vi "DATAreader5.vi"(6 "manual ADC rate, kHz":dbl=625.0, 7 "data info template":refnum<vi>, 10 "Cluster":cluster{"howmany":i16, "auto/man.":bool}={"howmany"=1, "auto/man."=FALSE} {"howmany" min=1 max=2}) -> (0 "error out":errorcluster, 1 "manual ADC rate?":bool, 2 "ADC type":i32, 3 "source":T1={"data path"=["D:\\LV\\testData\\11_06_14\\10_36_14ch#1", "D:\\LV\\testData\\11_06_14\\10_36_14ch#2", "D:\\LV\\testData\\11_06_14\\10_36_14ch#3", "D:\\LV\\testData\\11_06_14\\10_36_14ch#4", "D:\\LV\\testData\\11_06_14\\10_36_14ch#5", "D:\\LV\\testData\\11_06_14\\10_36_14ch#6", "D:\\LV\\testData\\11_06_14\\10_36_14ch#7", "D:\\LV\\testData\\11_06_14\\10_36_14ch#8", "D:\\LV\\testData\\11_06_14\\10_36_14ch#9", "D:\\LV\\testData\\11_06_14\\10_36_14ch#10", "D:\\LV\\testData\\11_06_14\\10_36_14ch#11", "D:\\LV\\testData\\11_06_14\\10_36_14ch#12", "D:\\LV\\testData\\11_06_14\\10_36_14ch#13", "D:\\LV\\testData\\11_06_14\\10_36_14ch#14", "D:\\LV\\testData\\11_06_14\\10_36_14ch#15", "D:\\LV\\testData\\11_06_14\\10_36_14ch#16", "D:\\LV\\testData\\11_06_14\\10_36_14ch#17", "D:\\LV\\testData\\11_06_14\\10_36_14ch#18", "D:\\LV\\testData\\11_06_14\\10_36_14ch#19", "D:\\LV\\testData\\11_06_14\\10_36_14ch#20", "D:\\LV\\testData\\11_06_14\\10_36_14ch#21", "D:\\LV\\testData\\11_06_14\\10_36_14ch#22", "D:\\LV\\testData\\11_06_14\\10_36_14ch#23", "D:\\LV\\testData\\11_06_14\\10_36_14ch#24", "D:\\LV\\testData\\11_06_14\\10_36_14ch#25", "D:\\LV\\testData\\11_06_14\\10_36_14ch#26", "D:\\LV\\testData\\11_06_14\\10_36_14ch#27", "D:\\LV\\testData\\11_06_14\\10_36_14ch#28", "D:\\LV\\testData\\11_06_14\\10_36_14ch#29", "D:\\LV\\testData\\11_06_14\\10_36_14ch#30"], "data"=[{"t0"=timestamp(0 s since 1904-01-01), "dt"=0.00015000000000000001, "Y"=array[600 elements], "attributes"=variant("source"=variant(cluster{"data path":string, "ADCintercadr_s":dbl, "data info":cluster{"probe name":string, "signal type":string, "Unit":string, "variable":string, "amplific.":dbl, "use or not *.info.txt?":i16, "U cascade, kV":string, "attenuation":dbl, "probe area, cm2":dbl, "plasma, a.m.u.":dbl}} {"data path"="D:\\LV\\testData\\11_06_14\\10_36_14ch#1", "ADCintercadr_s"=5e-06, "data info"={"probe name"="", "signal type"="", "Unit"="", "variable"="", "amplific."=0.0, "use or not *.info.txt?"=0, "U cascade, kV"="", "attenuation"=0.0, "probe area, cm2"=0.0, "plasma, a.m.u."=0.0}}))}, {"t0"=timestamp(4.999999999999959e-06 s since 1904-01-01), "dt"=0.00015000000000000001, "Y"=array[600 elements], "attributes"=variant("source"=variant(cluster{"data path":string, "ADCintercadr_s":dbl, "data info":cluster{"probe name":string, "signal type":string, "Unit":string, "variable":string, "amplific.":dbl, "use or not *.info.txt?":i16, "U cascade, kV":string, "attenuation":dbl, "probe area, cm2":dbl, "plasma, a.m.u.":dbl}} {"data path"="D:\\LV\\testData\\11_06_14\\10_36_14ch#2", "ADCintercadr_s"=5e-06, "data info"={"probe name"="", "signal type"="", "Unit"="", "variable"="", "amplific."=0.0, "use or not *.info.txt?"=0, "U cascade, kV"="", "attenuation"=0.0, "probe area, cm2"=0.0, "plasma, a.m.u."=0.0}}))}, {"t0"=timestamp(9.999999999999972e-06 s since 1904-01-01), "dt"=0.00015000000000000001, "Y"=array[600 elements], "attributes"=variant("source"=variant(cluster{"data path":string, "ADCintercadr_s":dbl, "data info":cluster{"probe name":string, "signal type":string, "Unit":string, "variable":string, "amplific.":dbl, "use or not *.info.txt?":i16, "U cascade, kV":string, "attenuation":dbl, "probe area, cm2":dbl, "plasma, a.m.u.":dbl}} {"data path"="D:\\LV\\testData\\11_06_14\\10_36_14ch#3", "ADCintercadr_s"=5e-06, "data info"={"probe name"="", "signal type"="", "Unit"="", "variable"="", "amplific."=0.0, "use or not *.info.txt?"=0, "U cascade, kV"="", "attenuation"=0.0, "probe area, cm2"=0.0, "plasma, a.m.u."=0.0}}))}, {"t0"=timestamp(1.4999999999999985e-05 s since 1904-01-01), "dt"=0.00015000000000000001, "Y"=array[600 elements], "attributes"=variant("source"=variant(cluster{"data path":string, "ADCintercadr_s":dbl, "data info":cluster{"probe name":string, "signal type":string, "Unit":string, "variable":string, "amplific.":dbl, "use or not *.info.txt?":i16, "U cascade, kV":string, "attenuation":dbl, "probe area, cm2":dbl, "plasma, a.m.u.":dbl}} {"data path"="D:\\LV\\testData\\11_06_14\\10_36_14ch#4", "ADCintercadr_s"=5e-06, "data info"={"probe name"="", "signal type"="", "Unit"="", "variable"="", "amplific."=0.0, "use or not *.info.txt?"=0, "U cascade, kV"="", "attenuation"=0.0, "probe area, cm2"=0.0, "plasma, a.m.u."=0.0}}))}, {"t0"=timestamp(1.9999999999999998e-05 s since 1904-01-01), "dt"=0.00015000000000000001, "Y"=array[600 elements], "attributes"=variant("source"=variant(cluster{"data path":string, "ADCintercadr_s":dbl, "data info":cluster{"probe name":string, "signal type":string, "Unit":string, "variable":string, "amplific.":dbl, "use or not *.info.txt?":i16, "U cascade, kV":string, "attenuation":dbl, "probe area, cm2":dbl, "plasma, a.m.u.":dbl}} {"data path"="D:\\LV\\testData\\11_06_14\\10_36_14ch#5", "ADCintercadr_s"=5e-06, "data info"={"probe name"="", "signal type"="", "Unit"="", "variable"="", "amplific."=0.0, "use or not *.info.txt?"=0, "U cascade, kV"="", "attenuation"=0.0, "probe area, cm2"=0.0, "plasma, a.m.u."=0.0}}))}, {"t0"=timestamp(2.4999999999999957e-05 s since 1904-01-01), "dt"=0.00015000000000000001, "Y"=array[600 elements], "attributes"=variant("source"=variant(cluster{"data path":string, "ADCintercadr_s":dbl, "data info":cluster{"probe name":string, "signal type":string, "Unit":string, "variable":string, "amplific.":dbl, "use or not *.info.txt?":i16, "U cascade, kV":string, "attenuation":dbl, "probe area, cm2":dbl, "plasma, a.m.u.":dbl}} {"data path"="D:\\LV\\testData\\11_06_14\\10_36_14ch#6", "ADCintercadr_s"=5e-06, "data info"={"probe name"="", "signal type"="", "Unit"="", "variable"="", "amplific."=0.0, "use or not *.info.txt?"=0, "U cascade, kV"="", "attenuation"=0.0, "probe area, cm2"=0.0, "plasma, a.m.u."=0.0}}))}, {"t0"=timestamp(2.999999999999997e-05 s since 1904-01-01), "dt"=0.00015000000000000001, "Y"=array[600 elements], "attributes"=variant("source"=variant(cluster{"data path":string, "ADCintercadr_s":dbl, "data info":cluster{"probe name":string, "signal type":string, "Unit":string, "variable":string, "amplific.":dbl, "use or not *.info.txt?":i16, "U cascade, kV":string, "attenuation":dbl, "probe area, cm2":dbl, "plasma, a.m.u.":dbl}} {"data path"="D:\\LV\\testData\\11_06_14\\10_36_14ch#7", "ADCintercadr_s"=5e-06, "data info"={"probe name"="", "signal type"="", "Unit"="", "variable"="", "amplific."=0.0, "use or not *.info.txt?"=0, "U cascade, kV"="", "attenuation"=0.0, "probe area, cm2"=0.0, "plasma, a.m.u."=0.0}}))}, {"t0"=timestamp(3.499999999999998e-05 s since 1904-01-01), "dt"=0.00015000000000000001, "Y"=array[600 elements], "attributes"=variant("source"=variant(cluster{"data path":string, "ADCintercadr_s":dbl, "data info":cluster{"probe name":string, "signal type":string, "Unit":string, "variable":string, "amplific.":dbl, "use or not *.info.txt?":i16, "U cascade, kV":string, "attenuation":dbl, "probe area, cm2":dbl, "plasma, a.m.u.":dbl}} {"data path"="D:\\LV\\testData\\11_06_14\\10_36_14ch#8", "ADCintercadr_s"=5e-06, "data info"={"probe name"="", "signal type"="", "Unit"="", "variable"="", "amplific."=0.0, "use or not *.info.txt?"=0, "U cascade, kV"="", "attenuation"=0.0, "probe area, cm2"=0.0, "plasma, a.m.u."=0.0}}))}, {"t0"=timestamp(3.9999999999999996e-05 s since 1904-01-01), "dt"=0.00015000000000000001, "Y"=array[600 elements], "attributes"=variant("source"=variant(cluster{"data path":string, "ADCintercadr_s":dbl, "data info":cluster{"probe name":string, "signal type":string, "Unit":string, "variable":string, "amplific.":dbl, "use or not *.info.txt?":i16, "U cascade, kV":string, "attenuation":dbl, "probe area, cm2":dbl, "plasma, a.m.u.":dbl}} {"data path"="D:\\LV\\testData\\11_06_14\\10_36_14ch#9", "ADCintercadr_s"=5e-06, "data info"={"probe name"="", "signal type"="", "Unit"="", "variable"="", "amplific."=0.0, "use or not *.info.txt?"=0, "U cascade, kV"="", "attenuation"=0.0, "probe area, cm2"=0.0, "plasma, a.m.u."=0.0}}))}, {"t0"=timestamp(4.4999999999999955e-05 s since 1904-01-01), "dt"=0.00015000000000000001, "Y"=array[600 elements], "attributes"=variant("source"=variant(cluster{"data path":string, "ADCintercadr_s":dbl, "data info":cluster{"probe name":string, "signal type":string, "Unit":string, "variable":string, "amplific.":dbl, "use or not *.info.txt?":i16, "U cascade, kV":string, "attenuation":dbl, "probe area, cm2":dbl, "plasma, a.m.u.":dbl}} {"data path"="D:\\LV\\testData\\11_06_14\\10_36_14ch#10", "ADCintercadr_s"=5e-06, "data info"={"probe name"="", "signal type"="", "Unit"="", "variable"="", "amplific."=0.0, "use or not *.info.txt?"=0, "U cascade, kV"="", "attenuation"=0.0, "probe area, cm2"=0.0, "plasma, a.m.u."=0.0}}))}, {"t0"=timestamp(4.999999999999997e-05 s since 1904-01-01), "dt"=0.00015000000000000001, "Y"=array[600 elements], "attributes"=variant("source"=variant(cluster{"data path":string, "ADCintercadr_s":dbl, "data info":cluster{"probe name":string, "signal type":string, "Unit":string, "variable":string, "amplific.":dbl, "use or not *.info.txt?":i16, "U cascade, kV":string, "attenuation":dbl, "probe area, cm2":dbl, "plasma, a.m.u.":dbl}} {"data path"="D:\\LV\\testData\\11_06_14\\10_36_14ch#11", "ADCintercadr_s"=5e-06, "data info"={"probe name"="", "signal type"="", "Unit"="", "variable"="", "amplific."=0.0, "use or not *.info.txt?"=0, "U cascade, kV"="", "attenuation"=0.0, "probe area, cm2"=0.0, "plasma, a.m.u."=0.0}}))}, {"t0"=timestamp(5.499999999999998e-05 s since 1904-01-01), "dt"=0.00015000000000000001, "Y"=array[600 elements], "attributes"=variant("source"=variant(cluster{"data path":string, "ADCintercadr_s":dbl, "data info":cluster{"probe name":string, "signal type":string, "Unit":string, "variable":string, "amplific.":dbl, "use or not *.info.txt?":i16, "U cascade, kV":string, "attenuation":dbl, "probe area, cm2":dbl, "plasma, a.m.u.":dbl}} {"data path"="D:\\LV\\testData\\11_06_14\\10_36_14ch#12", "ADCintercadr_s"=5e-06, "data info"={"probe name"="", "signal type"="", "Unit"="", "variable"="", "amplific."=0.0, "use or not *.info.txt?"=0, "U cascade, kV"="", "attenuation"=0.0, "probe area, cm2"=0.0, "plasma, a.m.u."=0.0}}))}, {"t0"=timestamp(5.9999999999999995e-05 s since 1904-01-01), "dt"=0.00015000000000000001, "Y"=array[600 elements], "attributes"=variant("source"=variant(cluster{"data path":string, "ADCintercadr_s":dbl, "data info":cluster{"probe name":string, "signal type":string, "Unit":string, "variable":string, "amplific.":dbl, "use or not *.info.txt?":i16, "U cascade, kV":string, "attenuation":dbl, "probe area, cm2":dbl, "plasma, a.m.u.":dbl}} {"data path"="D:\\LV\\testData\\11_06_14\\10_36_14ch#13", "ADCintercadr_s"=5e-06, "data info"={"probe name"="", "signal type"="", "Unit"="", "variable"="", "amplific."=0.0, "use or not *.info.txt?"=0, "U cascade, kV"="", "attenuation"=0.0, "probe area, cm2"=0.0, "plasma, a.m.u."=0.0}}))}, {"t0"=timestamp(6.500000000000001e-05 s since 1904-01-01), "dt"=0.00015000000000000001, "Y"=array[600 elements], "attributes"=variant("source"=variant(cluster{"data path":string, "ADCintercadr_s":dbl, "data info":cluster{"probe name":string, "signal type":string, "Unit":string, "variable":string, "amplific.":dbl, "use or not *.info.txt?":i16, "U cascade, kV":string, "attenuation":dbl, "probe area, cm2":dbl, "plasma, a.m.u.":dbl}} {"data path"="D:\\LV\\testData\\11_06_14\\10_36_14ch#14", "ADCintercadr_s"=5e-06, "data info"={"probe name"="", "signal type"="", "Unit"="", "variable"="", "amplific."=0.0, "use or not *.info.txt?"=0, "U cascade, kV"="", "attenuation"=0.0, "probe area, cm2"=0.0, "plasma, a.m.u."=0.0}}))}, {"t0"=timestamp(6.999999999999997e-05 s since 1904-01-01), "dt"=0.00015000000000000001, "Y"=array[600 elements], "attributes"=variant("source"=variant(cluster{"data path":string, "ADCintercadr_s":dbl, "data info":cluster{"probe name":string, "signal type":string, "Unit":string, "variable":string, "amplific.":dbl, "use or not *.info.txt?":i16, "U cascade, kV":string, "attenuation":dbl, "probe area, cm2":dbl, "plasma, a.m.u.":dbl}} {"data path"="D:\\LV\\testData\\11_06_14\\10_36_14ch#15", "ADCintercadr_s"=5e-06, "data info"={"probe name"="", "signal type"="", "Unit"="", "variable"="", "amplific."=0.0, "use or not *.info.txt?"=0, "U cascade, kV"="", "attenuation"=0.0, "probe area, cm2"=0.0, "plasma, a.m.u."=0.0}}))}, {"t0"=timestamp(7.499999999999998e-05 s since 1904-01-01), "dt"=0.00015000000000000001, "Y"=array[600 elements], "attributes"=variant("source"=variant(cluster{"data path":string, "ADCintercadr_s":dbl, "data info":cluster{"probe name":string, "signal type":string, "Unit":string, "variable":string, "amplific.":dbl, "use or not *.info.txt?":i16, "U cascade, kV":string, "attenuation":dbl, "probe area, cm2":dbl, "plasma, a.m.u.":dbl}} {"data path"="D:\\LV\\testData\\11_06_14\\10_36_14ch#16", "ADCintercadr_s"=5e-06, "data info"={"probe name"="", "signal type"="", "Unit"="", "variable"="", "amplific."=0.0, "use or not *.info.txt?"=0, "U cascade, kV"="", "attenuation"=0.0, "probe area, cm2"=0.0, "plasma, a.m.u."=0.0}}))}, {"t0"=timestamp(7.999999999999999e-05 s since 1904-01-01), "dt"=0.00015000000000000001, "Y"=array[600 elements], "attributes"=variant("source"=variant(cluster{"data path":string, "ADCintercadr_s":dbl, "data info":cluster{"probe name":string, "signal type":string, "Unit":string, "variable":string, "amplific.":dbl, "use or not *.info.txt?":i16, "U cascade, kV":string, "attenuation":dbl, "probe area, cm2":dbl, "plasma, a.m.u.":dbl}} {"data path"="D:\\LV\\testData\\11_06_14\\10_36_14ch#17", "ADCintercadr_s"=5e-06, "data info"={"probe name"="", "signal type"="", "Unit"="", "variable"="", "amplific."=0.0, "use or not *.info.txt?"=0, "U cascade, kV"="", "attenuation"=0.0, "probe area, cm2"=0.0, "plasma, a.m.u."=0.0}}))}, {"t0"=timestamp(8.5e-05 s since 1904-01-01), "dt"=0.00015000000000000001, "Y"=array[600 elements], "attributes"=variant("source"=variant(cluster{"data path":string, "ADCintercadr_s":dbl, "data info":cluster{"probe name":string, "signal type":string, "Unit":string, "variable":string, "amplific.":dbl, "use or not *.info.txt?":i16, "U cascade, kV":string, "attenuation":dbl, "probe area, cm2":dbl, "plasma, a.m.u.":dbl}} {"data path"="D:\\LV\\testData\\11_06_14\\10_36_14ch#18", "ADCintercadr_s"=5e-06, "data info"={"probe name"="", "signal type"="", "Unit"="", "variable"="", "amplific."=0.0, "use or not *.info.txt?"=0, "U cascade, kV"="", "attenuation"=0.0, "probe area, cm2"=0.0, "plasma, a.m.u."=0.0}}))}, {"t0"=timestamp(8.999999999999997e-05 s since 1904-01-01), "dt"=0.00015000000000000001, "Y"=array[600 elements], "attributes"=variant("source"=variant(cluster{"data path":string, "ADCintercadr_s":dbl, "data info":cluster{"probe name":string, "signal type":string, "Unit":string, "variable":string, "amplific.":dbl, "use or not *.info.txt?":i16, "U cascade, kV":string, "attenuation":dbl, "probe area, cm2":dbl, "plasma, a.m.u.":dbl}} {"data path"="D:\\LV\\testData\\11_06_14\\10_36_14ch#19", "ADCintercadr_s"=5e-06, "data info"={"probe name"="", "signal type"="", "Unit"="", "variable"="", "amplific."=0.0, "use or not *.info.txt?"=0, "U cascade, kV"="", "attenuation"=0.0, "probe area, cm2"=0.0, "plasma, a.m.u."=0.0}}))}, {"t0"=timestamp(9.499999999999998e-05 s since 1904-01-01), "dt"=0.00015000000000000001, "Y"=array[600 elements], "attributes"=variant("source"=variant(cluster{"data path":string, "ADCintercadr_s":dbl, "data info":cluster{"probe name":string, "signal type":string, "Unit":string, "variable":string, "amplific.":dbl, "use or not *.info.txt?":i16, "U cascade, kV":string, "attenuation":dbl, "probe area, cm2":dbl, "plasma, a.m.u.":dbl}} {"data path"="D:\\LV\\testData\\11_06_14\\10_36_14ch#20", "ADCintercadr_s"=5e-06, "data info"={"probe name"="", "signal type"="", "Unit"="", "variable"="", "amplific."=0.0, "use or not *.info.txt?"=0, "U cascade, kV"="", "attenuation"=0.0, "probe area, cm2"=0.0, "plasma, a.m.u."=0.0}}))}, {"t0"=timestamp(9.999999999999999e-05 s since 1904-01-01), "dt"=0.00015000000000000001, "Y"=array[600 elements], "attributes"=variant("source"=variant(cluster{"data path":string, "ADCintercadr_s":dbl, "data info":cluster{"probe name":string, "signal type":string, "Unit":string, "variable":string, "amplific.":dbl, "use or not *.info.txt?":i16, "U cascade, kV":string, "attenuation":dbl, "probe area, cm2":dbl, "plasma, a.m.u.":dbl}} {"data path"="D:\\LV\\testData\\11_06_14\\10_36_14ch#21", "ADCintercadr_s"=5e-06, "data info"={"probe name"="", "signal type"="", "Unit"="", "variable"="", "amplific."=0.0, "use or not *.info.txt?"=0, "U cascade, kV"="", "attenuation"=0.0, "probe area, cm2"=0.0, "plasma, a.m.u."=0.0}}))}, {"t0"=timestamp(0.000105 s since 1904-01-01), "dt"=0.00015000000000000001, "Y"=array[600 elements], "attributes"=variant("source"=variant(cluster{"data path":string, "ADCintercadr_s":dbl, "data info":cluster{"probe name":string, "signal type":string, "Unit":string, "variable":string, "amplific.":dbl, "use or not *.info.txt?":i16, "U cascade, kV":string, "attenuation":dbl, "probe area, cm2":dbl, "plasma, a.m.u.":dbl}} {"data path"="D:\\LV\\testData\\11_06_14\\10_36_14ch#22", "ADCintercadr_s"=5e-06, "data info"={"probe name"="", "signal type"="", "Unit"="", "variable"="", "amplific."=0.0, "use or not *.info.txt?"=0, "U cascade, kV"="", "attenuation"=0.0, "probe area, cm2"=0.0, "plasma, a.m.u."=0.0}}))}, {"t0"=timestamp(0.00010999999999999996 s since 1904-01-01), "dt"=0.00015000000000000001, "Y"=array[600 elements], "attributes"=variant("source"=variant(cluster{"data path":string, "ADCintercadr_s":dbl, "data info":cluster{"probe name":string, "signal type":string, "Unit":string, "variable":string, "amplific.":dbl, "use or not *.info.txt?":i16, "U cascade, kV":string, "attenuation":dbl, "probe area, cm2":dbl, "plasma, a.m.u.":dbl}} {"data path"="D:\\LV\\testData\\11_06_14\\10_36_14ch#23", "ADCintercadr_s"=5e-06, "data info"={"probe name"="", "signal type"="", "Unit"="", "variable"="", "amplific."=0.0, "use or not *.info.txt?"=0, "U cascade, kV"="", "attenuation"=0.0, "probe area, cm2"=0.0, "plasma, a.m.u."=0.0}}))}, {"t0"=timestamp(0.00011499999999999998 s since 1904-01-01), "dt"=0.00015000000000000001, "Y"=array[600 elements], "attributes"=variant("source"=variant(cluster{"data path":string, "ADCintercadr_s":dbl, "data info":cluster{"probe name":string, "signal type":string, "Unit":string, "variable":string, "amplific.":dbl, "use or not *.info.txt?":i16, "U cascade, kV":string, "attenuation":dbl, "probe area, cm2":dbl, "plasma, a.m.u.":dbl}} {"data path"="D:\\LV\\testData\\11_06_14\\10_36_14ch#24", "ADCintercadr_s"=5e-06, "data info"={"probe name"="", "signal type"="", "Unit"="", "variable"="", "amplific."=0.0, "use or not *.info.txt?"=0, "U cascade, kV"="", "attenuation"=0.0, "probe area, cm2"=0.0, "plasma, a.m.u."=0.0}}))}, {"t0"=timestamp(0.00011999999999999999 s since 1904-01-01), "dt"=0.00015000000000000001, "Y"=array[600 elements], "attributes"=variant("source"=variant(cluster{"data path":string, "ADCintercadr_s":dbl, "data info":cluster{"probe name":string, "signal type":string, "Unit":string, "variable":string, "amplific.":dbl, "use or not *.info.txt?":i16, "U cascade, kV":string, "attenuation":dbl, "probe area, cm2":dbl, "plasma, a.m.u.":dbl}} {"data path"="D:\\LV\\testData\\11_06_14\\10_36_14ch#25", "ADCintercadr_s"=5e-06, "data info"={"probe name"="", "signal type"="", "Unit"="", "variable"="", "amplific."=0.0, "use or not *.info.txt?"=0, "U cascade, kV"="", "attenuation"=0.0, "probe area, cm2"=0.0, "plasma, a.m.u."=0.0}}))}, {"t0"=timestamp(0.000125 s since 1904-01-01), "dt"=0.00015000000000000001, "Y"=array[600 elements], "attributes"=variant("source"=variant(cluster{"data path":string, "ADCintercadr_s":dbl, "data info":cluster{"probe name":string, "signal type":string, "Unit":string, "variable":string, "amplific.":dbl, "use or not *.info.txt?":i16, "U cascade, kV":string, "attenuation":dbl, "probe area, cm2":dbl, "plasma, a.m.u.":dbl}} {"data path"="D:\\LV\\testData\\11_06_14\\10_36_14ch#26", "ADCintercadr_s"=5e-06, "data info"={"probe name"="", "signal type"="", "Unit"="", "variable"="", "amplific."=0.0, "use or not *.info.txt?"=0, "U cascade, kV"="", "attenuation"=0.0, "probe area, cm2"=0.0, "plasma, a.m.u."=0.0}}))}, {"t0"=timestamp(0.00013000000000000002 s since 1904-01-01), "dt"=0.00015000000000000001, "Y"=array[600 elements], "attributes"=variant("source"=variant(cluster{"data path":string, "ADCintercadr_s":dbl, "data info":cluster{"probe name":string, "signal type":string, "Unit":string, "variable":string, "amplific.":dbl, "use or not *.info.txt?":i16, "U cascade, kV":string, "attenuation":dbl, "probe area, cm2":dbl, "plasma, a.m.u.":dbl}} {"data path"="D:\\LV\\testData\\11_06_14\\10_36_14ch#27", "ADCintercadr_s"=5e-06, "data info"={"probe name"="", "signal type"="", "Unit"="", "variable"="", "amplific."=0.0, "use or not *.info.txt?"=0, "U cascade, kV"="", "attenuation"=0.0, "probe area, cm2"=0.0, "plasma, a.m.u."=0.0}}))}, {"t0"=timestamp(0.00013499999999999997 s since 1904-01-01), "dt"=0.00015000000000000001, "Y"=array[600 elements], "attributes"=variant("source"=variant(cluster{"data path":string, "ADCintercadr_s":dbl, "data info":cluster{"probe name":string, "signal type":string, "Unit":string, "variable":string, "amplific.":dbl, "use or not *.info.txt?":i16, "U cascade, kV":string, "attenuation":dbl, "probe area, cm2":dbl, "plasma, a.m.u.":dbl}} {"data path"="D:\\LV\\testData\\11_06_14\\10_36_14ch#28", "ADCintercadr_s"=5e-06, "data info"={"probe name"="", "signal type"="", "Unit"="", "variable"="", "amplific."=0.0, "use or not *.info.txt?"=0, "U cascade, kV"="", "attenuation"=0.0, "probe area, cm2"=0.0, "plasma, a.m.u."=0.0}}))}, {"t0"=timestamp(0.00014 s since 1904-01-01), "dt"=0.00015000000000000001, "Y"=array[600 elements], "attributes"=variant("source"=variant(cluster{"data path":string, "ADCintercadr_s":dbl, "data info":cluster{"probe name":string, "signal type":string, "Unit":string, "variable":string, "amplific.":dbl, "use or not *.info.txt?":i16, "U cascade, kV":string, "attenuation":dbl, "probe area, cm2":dbl, "plasma, a.m.u.":dbl}} {"data path"="D:\\LV\\testData\\11_06_14\\10_36_14ch#29", "ADCintercadr_s"=5e-06, "data info"={"probe name"="", "signal type"="", "Unit"="", "variable"="", "amplific."=0.0, "use or not *.info.txt?"=0, "U cascade, kV"="", "attenuation"=0.0, "probe area, cm2"=0.0, "plasma, a.m.u."=0.0}}))}, {"t0"=timestamp(0.000145 s since 1904-01-01), "dt"=0.00015000000000000001, "Y"=array[600 elements], "attributes"=variant("source"=variant(cluster{"data path":string, "ADCintercadr_s":dbl, "data info":cluster{"probe name":string, "signal type":string, "Unit":string, "variable":string, "amplific.":dbl, "use or not *.info.txt?":i16, "U cascade, kV":string, "attenuation":dbl, "probe area, cm2":dbl, "plasma, a.m.u.":dbl}} {"data path"="D:\\LV\\testData\\11_06_14\\10_36_14ch#30", "ADCintercadr_s"=5e-06, "data info"={"probe name"="", "signal type"="", "Unit"="", "variable"="", "amplific."=0.0, "use or not *.info.txt?"=0, "U cascade, kV"="", "attenuation"=0.0, "probe area, cm2"=0.0, "plasma, a.m.u."=0.0}}))}]}, 4 "chan.in.files":i16[](array[numeric]), 11 "ADC gain applied from *.par":bool)   [LabVIEW 2014]
uses:
  <vilib>/Waveform/WDTOps.llb/WDT Number of Waveform Samples DBL.vi
panel:
  out "txt data rate":dbl[](array[numeric])
  out "allpathes":path[](array[path])
  out "Array":string[](array[string])
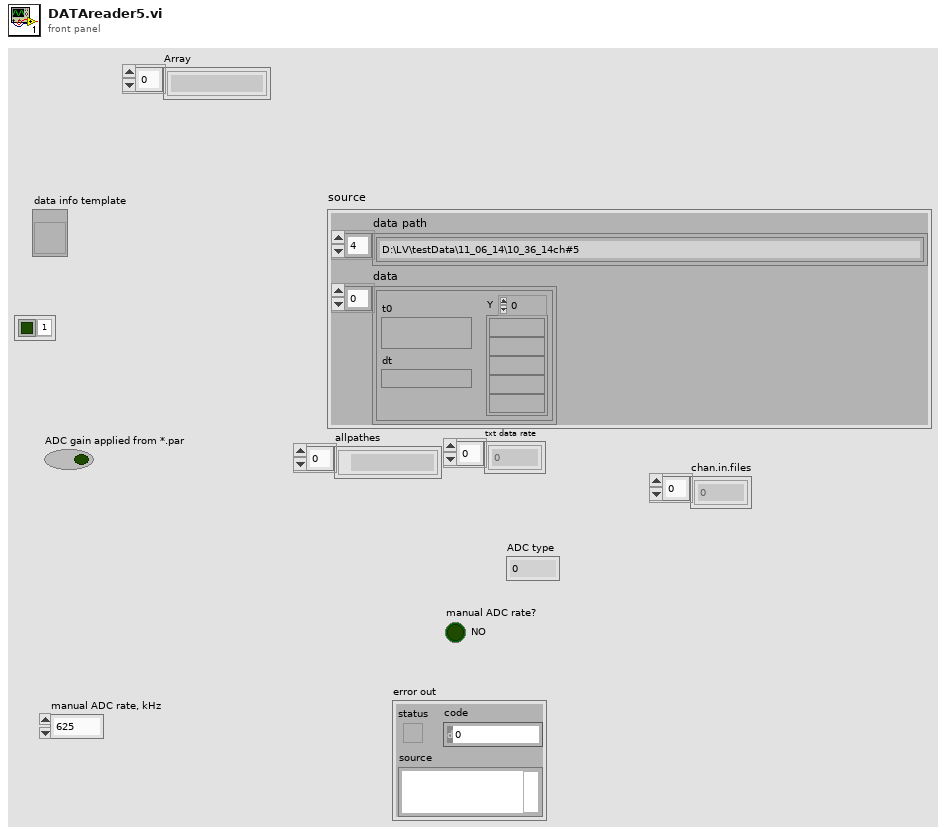
[diagram p1: front panel]
types:
  T1 = cluster{"data path":string[], "data":waveform(dbl)[]}
  T2 = enum16{"open", "replace", "create", "open or create", "replace or create", "replace or create with confirmation"}
  T3 = enum16{"deny read/write", "deny write-only", "deny none"}
  T4 = enum16{"big-endian, network order", "native, host order", "little-endian"}
  T5 = cluster{" CodeString":string, "DeviceName":string, "TimeString":string, "ChannelsMax":i16, "RealChannelsQuantity":i16, "RealKadrsQuantity":i64, "RealSamplesQuantity":i64, "TotalTime (sec) - long double in new *.par !!":string, "AdcRate (kHz)":dbl, "InterkadrDelay (ms)":dbl, "ChannelRate (kHz)":dbl, "ActiveAdcChannelArray":u32[], "AdcChannelArray":u8[], "AdcGainArray":u8[], "IsSignalArray":u8[], "DataFormat":i32, "RealKadrs64":i64, "AdcScale":dbl[], "AdcOffset":dbl[], "channel_name":string[], "LastModified":string}
  T6 = cluster{"data path":string, "ADCintercadr_s":dbl, "data info":cluster{"use or not *.info.txt?":i16, "probe name":string, "signal type":string, "Unit":string, "variable":string, "attenuation factor":dbl, "amplification factor":dbl, "extracoef#1":dbl, "extracoef#2":dbl, "U cascade, kV":string, "probe area, cm2":dbl, "plasma, a.m.u.":dbl}, "channel_name":string, "channels_in_file":i32, "LastModified":string}
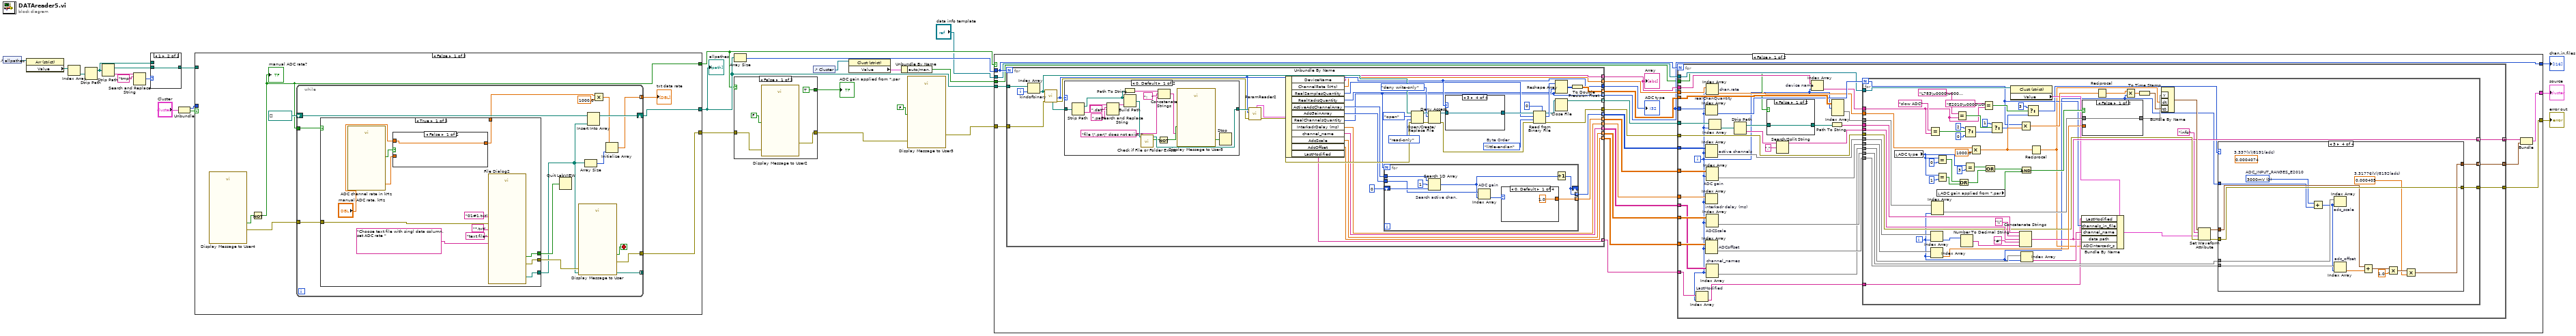
[diagram p0: block diagram]
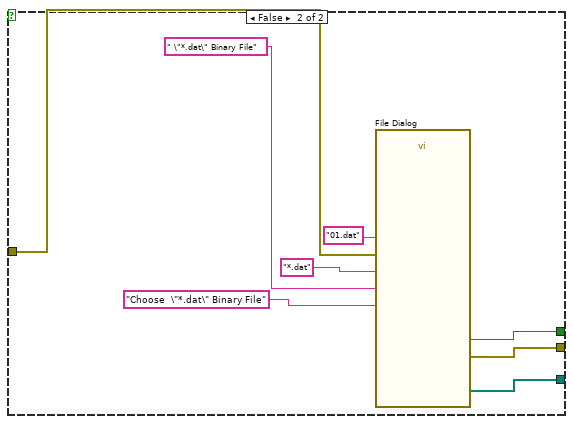
[diagram p4: hidden frame]
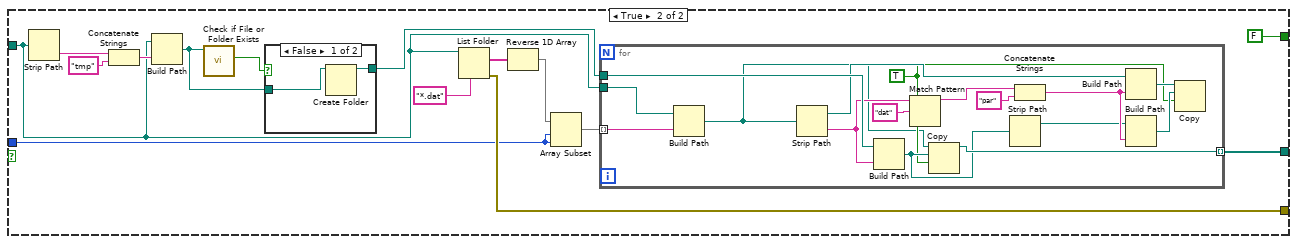
[diagram p5: hidden frame]
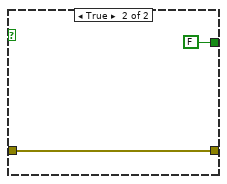
[diagram p7: hidden frame]
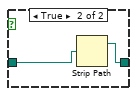
[diagram p8: hidden frame]
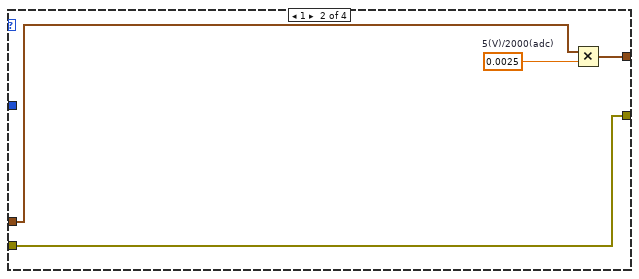
[diagram p10: hidden frame]
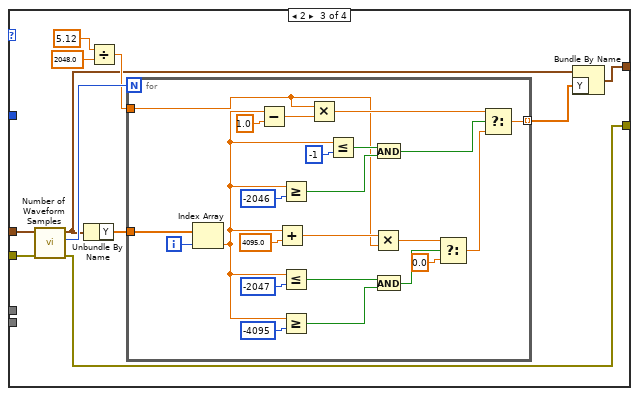
[diagram p11: hidden frame]
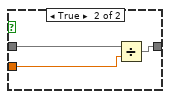
[diagram p12: hidden frame]
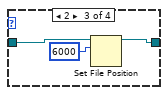
[diagram p16: hidden frame]
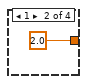
[diagram p17: hidden frame]
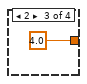
[diagram p18: hidden frame]
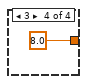
[diagram p19: hidden frame]
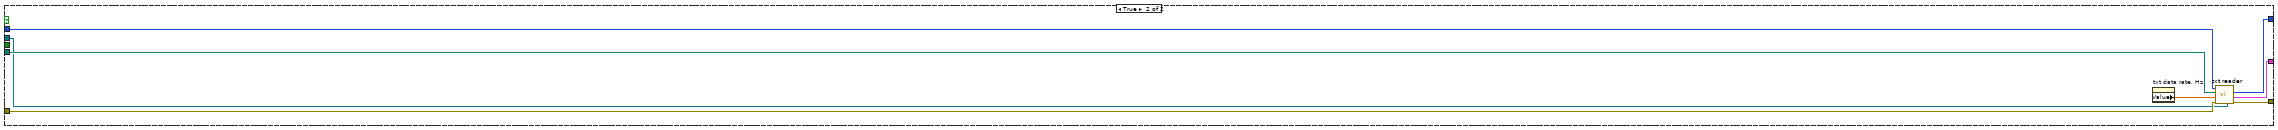
[diagram p20: hidden frame]
diagram:
  n1 = control-ref of="allpathes"() -> (w13:refnum<vi>)
  n2 = property class="Arr (strict)"(reference=w13) -> ("Value"=w12:path[])  [unwired: 1 in, 2 out]
  n3 = Index Array(array=w12) -> (element=w3:path)  [unwired: 1 in]
  n4 = Strip Path(path=w3) -> (stripped path=w6:path)  [unwired: 1 out]
  n5 = Strip Path(path=w6) -> (stripped path=w5:path, name=w8:string)
  n6 = Search and Replace String(input string=w8, search string="tmp") -> (number of replacements=w7:i32)  [unwired: 6 in, 3 out]
  n7 = case shown="1" w7 {
    tunnel: w6 -> [w28 _]
    tunnel: [w28 w29] -> w2
    tunnel: w5 -> [_ w29]
    frame 0, Default {
    }
    frame 1 {
    }
  }
  n8 = Unbundle("Cluster") -> ("howmany"=w14:i16, "auto/man."=w15:bool)
  n9 = case shown="False" w15 {
    tunnel: [w36 w76] -> w24
    tunnel: [w30 w78] -> w22
    tunnel: [w32 FALSE ("txt")] -> w18
    tunnel: w14 -> [_ w73]
    tunnel: w2 -> [_ w74]
    frame False {
      n10 = call "Display Message to User4"() -> ("error out"=w34:errorcluster, "binary"=w33:bool)  [unwired: 10 in]
      n11 = Not(x=w33) -> (.not. x?=w32:bool)
      "manual ADC rate?" <- w32
      n12 = while {
        tunnel: [w50] -> w36
        tunnel: w32 -> [w48]
        shift-right: [w47] -> w30
        shift-left: path[] [] -> [w45]
        tunnel: w34 -> [w43]
        tunnel: [w39] -> _ mode=concatenating
        tunnel: [w37] -> w31 mode=concatenating
        stop <- w44 stop-if-true
        n13 = case shown="True" w48 {
          tunnel: [w60 w69] -> w46
          tunnel: [w59 w68] -> w49
          tunnel: [w57 w66] -> w39
          tunnel: w43 -> [w55 w65]
          tunnel: [w51 _] -> w41
          frame True {
            n14 = call "ADC channel rate in kHz"() -> ("ADC channel rate, kHz"=w54:dbl, "OK"=w53:bool)  [unwired: 17 in, 1 out]
            n15 = case shown="False" w53 {
              tunnel: w54 -> [_ w64]
              tunnel: "manual ADC rate, kHz" -> [w63 _]
              tunnel: [w63 w64] -> w51
              frame False {
              }
              frame True {
              }
            }
            n16 = call "File Dialog2"("prompt"="Choose text file with singl data column, set ADC rate " ("Prompt"), "default name"="01#1.txt", "error in"=w55, "pattern (all files)"="*.txt", "pattern label"="text file" ("Prompt")) -> ("selected paths"=w57:path[], "cancelled"=w60:bool, "error out"=w59:errorcluster)  [unwired: 7 in, 1 out]
          }
          frame False {
            n17 = call "File Dialog"("prompt"="Choose  \"*.dat\" Binary File" ("Prompt"), "default name"="01.dat", "error in"=w65, "pattern (all files)"="*.dat", "pattern label"=" \"*.dat\" Binary File" ("Prompt")) -> ("selected paths"=w66:path[], "cancelled"=w69:bool, "error out"=w68:errorcluster)  [unwired: 7 in, 1 out]
          }
        }
        n18 = Quit LabVIEW(quit? (T)=w46) -> ()
        n19 = call "Display Message to User"("error in (no error)"=w49) -> ("error out"=w50:errorcluster, "NO"=w44:bool)  [unwired: 9 in]
        n20 = Array Size(array=w39) -> (size(s)=w38:i32)
        n21 = Insert Into Array(array=w45, new element=w39) -> (w47:path[])  [unwired: 1 in]
        n22 = Multiply(x=w41, y=1000.0 ("manual ADC rate, kHz")) -> (x*y=w40:dbl)
        n23 = Initialize Array(w40, w38) -> (w37:dbl[])
      }
      "txt data rate" <- w31
    }
    frame True {
      n24 = Strip Path(path=w74) -> (name=w80:string)  [unwired: 1 out]
      n25 = Concatenate Strings(w80, "tmp" ("name or relative path")) -> (w83:string)
      n26 = Build Path(base path=w74, name or relative path=w83) -> (appended path=w82:path)
      n27 = call <vilib>:"Check if File or Folder Exists.vi"("path"=w82) -> ("file or folder exists?"=w85:bool)  [unwired: 8 in, 2 out]
      n28 = case shown="False" w85 {
        tunnel: w82 -> [w105 w106]
        tunnel: [w104 w106] -> w79
        frame False {
          n29 = Create Folder(path (use dialog)=w105) -> (created path=w104:path)  [unwired: 2 in, 2 out]
        }
        frame True {
        }
      }
      n30 = List Folder(path=w74, pattern="*.dat") -> (filenames=w75:string[], error out=w76:errorcluster)  [unwired: 2 in, 2 out]
      n31 = Reverse 1D Array(array=w75) -> (reversed array=w86:string[])
      n32 = Array Subset(array=w86, index=w73, length=w73) -> (w81:string[])
      n33 = for {
        tunnel: w81 -> [w90] mode=indexing
        tunnel: w79 -> [w103]
        tunnel: [w102] -> w78 mode=indexing
        tunnel: w74 -> [w89]
        w92 = TRUE ("overwrite (F)")
        n34 = Build Path(base path=w89, name or relative path=w90) -> (appended path=w88:path)
        n35 = Strip Path(path=w88) -> (stripped path=w101:path, name=w91:string)
        n36 = Build Path(base path=w103, name or relative path=w91) -> (appended path=w99:path)
        n37 = Match Pattern(string=w91, regular expression="dat") -> (before substring=w97:string)  [unwired: 1 in, 3 out]
        n38 = Copy(9:w92, 10:w99, 11:w88) -> (3:w102:path)  [unwired: 2 in, 2 out]
        n39 = Strip Path(path=w99) -> (stripped path=w94:path)  [unwired: 1 out]
        n40 = Concatenate Strings(w97, "par" ("name or relative path")) -> (w95:string)
        n41 = Build Path(base path=w101, name or relative path=w95) -> (appended path=w100:path)
        n42 = Build Path(base path=w94, name or relative path=w95) -> (appended path=w93:path)
        n43 = Copy(9:w92, 10:w93, 11:w100) -> ()  [unwired: 2 in, 3 out]
      }
    }
  }
  "allpathes" <- w22
  n44 = Array Size(array=w22) -> (size(s)=w26:i32)
  n45 = case shown="False" w18 {
    tunnel: [TRUE FALSE ("YES")] -> w20
    tunnel: w24 -> [w110 w111]
    tunnel: [w109 w111] -> w23
    frame False {
      n46 = call "Display Message to User2"("error in (no error)"=w110, "Enable"=FALSE) -> ("error out"=w109:errorcluster)  [unwired: 8 in, 1 out]
    }
    frame True {
    }
  }
  "ADC gain applied from *.par" <- w20
  n47 = control-ref of="Cluster"() -> (w11:refnum<vi>)
  n48 = property class="Clust (strict)"(reference=w11) -> ("Value"=w10:cluster{"howmany":i16, "auto/man.":bool})  [unwired: 1 in, 2 out]
  n49 = Unbundle By Name(w10) -> ("auto/man."=w9:bool)
  n50 = call "Display Message to User3"("error in (no error)"=w23, "Enable"=FALSE ("YES")) -> ("error out"=w25:errorcluster)  [unwired: 8 in, 1 out]
  n51 = case shown="False" w18 {
    tunnel: [w135 w374] -> w27
    tunnel: w22 -> [w134 w376]
    tunnel: w26 -> [w133 w377]
    tunnel: w25 -> [w126 w375]
    tunnel: [w121 w373] -> w19
    tunnel: "data info template" -> [w119 w372]
    tunnel: [w117 w371] -> w17
    tunnel: w9 -> [w116 _]
    frame False {
      n52 = for {
        N: w133 -> [_]
        tunnel: w126 -> [w310]
        tunnel: [w300] -> w117 mode=indexing
        tunnel: [w325] -> w127 mode=indexing
        tunnel: [w305] -> w128 mode=indexing
        tunnel: w134 -> [w324]
        tunnel: [w318] -> w129 mode=indexing
        tunnel: [w314] -> w130 mode=indexing
        tunnel: [w321] -> w132
        tunnel: [w320] -> w131 mode=indexing
        tunnel: [w308] -> w125
        tunnel: [w299] -> w124 mode=indexing
        tunnel: [w298] -> w120 mode=indexing
        tunnel: [w306] -> w118 mode=indexing
        tunnel: [w297] -> w115 mode=indexing
        tunnel: [w296] -> w114 mode=indexing
        tunnel: [w295] -> w113 mode=indexing
        i -> [w323]
        w334 = T4."little-endian"  # Byte Order
        n53 = Index Array(array=w324, index=w323) -> (element=w313:path)
        n54 = call "kindofbinary.vi"("error in (no error)"=w310, "selected \"*.dat\" path"=w313) -> ("error out"=w309:errorcluster, "what kind of binary"=w308:i32, "output path"=w312:path)  [unwired: 7 in]
        n55 = case shown="0, Default" w308 {
          tunnel: w312 -> [w346 w351]
          tunnel: [w345 w351] -> w311
          frame 0, Default {
            n56 = Strip Path(path=w346) -> (stripped path=w337:path, name=w350:string)
            n57 = Search and Replace String(input string=w350, search string=".dat", replace string=".par" ("replace string (\"\")")) -> (result string=w347:string)  [unwired: 5 in, 3 out]
            n58 = Path To String(path=w337) -> (string=w341:string)
            n59 = Build Path(base path=w337, name or relative path=w347) -> (appended path=w342:path)
            n60 = call <vilib>:"Check if File or Folder Exists.vi"("path"=w342) -> ("file or folder exists?"=w344:bool, "dup path"=w345:path)  [unwired: 8 in, 1 out]
            n61 = Not(x=w344) -> (.not. x?=w343:bool)
            n62 = Concatenate Strings(w341, ":   " ("string"), "file \".par\" does not exist !" ("string")) -> (w338:string)
            n63 = call "Display Message to User5"("Enable"=w343, "Message"=w338) -> ("OK"=w336:bool)  [unwired: 8 in, 1 out]
            n64 = Stop(stop? (T)=w336) -> ()
          }
          frame 2 {
          }
        }
        n65 = call "ParamReader2.vi"("error in (no error)"=w309, "what kind of binary"=w308, "selected path"=w311) -> ("error out"=w317:errorcluster, "Cluster"=w307:T5)  [unwired: 6 in, 1 out]
        n66 = Unbundle By Name(w307) -> ("DeviceName"=w306:string, "ChannelRate (kHz)"=w305:dbl, "RealSamplesQuantity"=w304:i64, "RealKadrsQuantity"=w303:i64, "ActiveAdcChannelArray"=w302:u32[], "AdcGainArray"=w301:u8[], "RealChannelsQuantity"=w300:i16, "InterkadrDelay (ms)"=w299:dbl, "channel_name"=w298:string[], "AdcScale"=w297:dbl[], "AdcOffset"=w296:dbl[], "LastModified"=w295:string)
        n67 = for {
          N: w300 -> [_]
          tunnel: w302 -> [w365]
          shift-right: [w358] -> _
          shift-left: 0 -> [w363]
          tunnel: w301 -> [w362]
          tunnel: [w360] -> w320 mode=indexing
          tunnel: [w358] -> w314 mode=indexing
          n68 = Search 1D Array "Search active chan."(1D array=w365, element=1, start index (0)=w363) -> (index of element=w359:i32)
          n69 = Index Array "ADC gain"(array=w362, index=w359) -> (element=w361:u8)
          n70 = case shown="0, Default" w361 {
            tunnel: [1.0 2.0 4.0 8.0] -> w360
            frame 0, Default {
            }
            frame 1 {
            }
            frame 2 {
            }
            frame 3 {
            }
          }
          n71 = Increment(x=w359) -> (x+1=w358:i32)
        }
        n72 = Open/Create/Replace File(file path (use dialog)=w313, error in=w317, operation (0:open)=T2."open", access (0:read/write)=enum16{"read/write", "read-only", "write-only"}."read-only") -> (refnum out=w332:refnum<file>, error out=w333:errorcluster)  [unwired: 2 in, 1 out]
        n73 = Deny Access(4:w333, 6:T3."deny write-only" ("deny mode (0:deny read/write)"), 7:w332) -> (0:w329:errorcluster, 3:w316:refnum<file>)
        n74 = case shown="3" w308 {
          tunnel: w316 -> [w352 w353 w355 w357]
          tunnel: [w352 w353 w354 w357] -> w315
          frame 0, Default {
          }
          frame 1 {
          }
          frame 2 {
            n75 = Set File Position(offset (in bytes) (0)=i64 6000, refnum=w355) -> (refnum out=w354:refnum<file>)  [unwired: 2 in, 1 out]
          }
          frame 3 {
          }
        }
        n76 = Read from Binary File(5:i16 0 ("count (1)"), 8:w329, 9:w334, 10:w304, 11:w315) -> (0:w321:errorcluster, 2:w327:i16[], 3:w319:refnum<file>)  [unwired: 1 in, 1 out]
        n77 = Reshape Array(w327, w303, w300) -> (w326:i16[][])
        n78 = Close File(refnum=w319) -> (path=w318:path)  [unwired: 1 in, 1 out]
        n79 = To Double Precision Float(number=w326) -> (double precision float=w325:dbl[][])
      }
      "ADC type" <- w125
      "Array" <- w118
      n80 = for {
        N: w133 -> [_]
        tunnel: w117 -> [w168]
        tunnel: w127 -> [w170]
        tunnel: w128 -> [w171]
        tunnel: w129 -> [w167]
        tunnel: w130 -> [w166]
        tunnel: w131 -> [w165]
        tunnel: [w163] -> w135
        tunnel: w132 -> [w162]
        tunnel: w124 -> [w156]
        tunnel: [w154] -> w122 mode=concatenating
        tunnel: [w153] -> w123 mode=concatenating
        tunnel: w120 -> [w140]
        tunnel: w119 -> [w150]
        tunnel: w118 -> [w149]
        tunnel: w116 -> [w147]
        tunnel: w115 -> [w144]
        tunnel: w114 -> [w143]
        tunnel: w113 -> [w138]
        i -> [w137]
        n81 = Index Array "LastModified"(array=w138, index=w137) -> (element=w136:string)
        n82 = Index Array "realChanQuantity"(array=w168, index=w137) -> (element=w152:i16)
        n83 = Index Array "active channels"(array=w166, index (row)=w137) -> (element=w161:i32[])  [unwired: 1 in]
        n84 = Index Array "interkadr delay (ms)"(array=w156, index=w137) -> ()  [unwired: 1 out]
        n85 = Index Array "ADCoffset"(array=w143, index (row)=w137) -> (element=w141:dbl[])  [unwired: 1 in]
        n86 = Index Array "chan.rate"(array=w171, index=w137) -> (element=w151:dbl)
        n87 = Index Array "ADCScale"(array=w144, index (row)=w137) -> (element=w142:dbl[])  [unwired: 1 in]
        n88 = Index Array "ADC gain"(array=w165, index (row)=w137) -> (element=w164:dbl[])  [unwired: 1 in]
        n89 = Index Array "channel_names"(array=w140, index (row)=w137) -> (element=w139:string[])  [unwired: 1 in]
        n90 = Index Array(array=w167, index=w137) -> (element=w160:path)
        n91 = Strip Path(path=w160) -> (stripped path=w146:path, name=w158:string)
        n92 = case shown="False" w147 {
          tunnel: w146 -> [w172 w174]
          tunnel: [w172 w173] -> w145
          frame False {
          }
          frame True {
            n93 = Strip Path(path=w174) -> (stripped path=w173:path)  [unwired: 1 out]
          }
        }
        n94 = Search/Split String(string=w158, search string/char (-)="." ("regular expression")) -> (substring before match=w157:string)  [unwired: 1 in, 2 out]
        n95 = Index Array "device name"(array=w149, index=w137) -> (element=w148:string)
        n96 = Path To String(path=w145) -> (string=w155:string)
        n97 = Index Array(array=w170, index (dim 0)=w137) -> (element=w169:dbl[][])  [unwired: 2 in]
        n98 = for {
          N: w152 -> [w181]
          tunnel: w169 -> [w237]
          tunnel: w151 -> [w180]
          tunnel: w164 -> [w235]
          tunnel: [w220] -> w163
          tunnel: w162 -> [w222]
          tunnel: w161 -> [w232]
          tunnel: w155 -> [w229]
          tunnel: w157 -> [w231]
          tunnel: [w211] -> w153 mode=indexing
          tunnel: [w212] -> w154 mode=indexing
          tunnel: w139 -> [w200]
          tunnel: w150 -> [w197]
          tunnel: w148 -> [w187]
          tunnel: w142 -> [w178]
          tunnel: w141 -> [w177]
          tunnel: w136 -> [w175]
          i -> [w176]
          n99 = local read "ADC type"() -> (w196:i32)
          n100 = Equal?(x="slow ADC", y=w187) -> (x = y?=w186:bool)
          n101 = Index Array(array=w232, index=w176) -> (element=w219:i32)
          n102 = Index Array(array=w235, index=w176) -> (element=w234:dbl)
          n103 = Index Array(array=w237, index (col)=w176) -> (element=w233:dbl[])  [unwired: 1 in]
          n104 = Equal?(x=w196, y=0) -> (x = y?=w217:bool)
          n105 = Equal?(x=w196, y=1) -> (x = y?=w215:bool)
          n106 = local read "ADC gain applied from *.par"() -> (w214:bool)
          n107 = Equal?(x="L783\u0000\u0000\u0000\u0000\u0000\u0000\u0000\u0000\u0000\u0000\u0000\u0000\u0000", y=w187) -> (x = y?=w190:bool)
          n108 = Or(x=w217, y=w215) -> (x .or. y?=w202:bool)
          n109 = Number To Decimal String(number=w219) -> (decimal integer string=w230:string)  [unwired: 1 in]
          n110 = Equal?(x=w196, y=3) -> (x = y?=w203:bool)
          n111 = Select(t=2, s=w186, f=0) -> (s? t:f=w184:i32)
          n112 = Multiply(x=w180, y=1000.0) -> (x*y=w207:dbl)
          n113 = Equal?(x="E2010\u0000\u0000\u0000\u0000\u0000\u0000\u0000\u0000\u0000\u0000\u0000\u0000", y=w187) -> (x = y?=w193:bool)
          n114 = Or(x=w203, y=w202) -> (x .or. y?=w201:bool)
          n115 = Select(t=1, s=w190, f=w184) -> (s? t:f=w183:i32)
          n116 = property on="Property Node" class="Clust (strict)"(reference=w197) -> ("Value"=w198:T6)  [unwired: 1 in, 2 out]
          n117 = Concatenate Strings(w229, "\\" ("string"), w231, "#" ("string"), w230) -> (w211:string)
          n118 = Multiply(x=w181, y=w207) -> (x*y=w206:dbl)
          n119 = And(x=w201, y=w214) -> (x .and. y?=w213:bool)
          n120 = Index Array(array=w200, index=w176) -> (element=w199:string)
          n121 = Select(t=3, s=w193, f=w183) -> (s? t:f=w192:i32)
          n122 = Reciprocal(x=w207) -> (1/x=w179:dbl)
          n123 = Bundle By Name(cluster=w198, "LastModified"=w175, "channels_in_file"=w181, "channel_name"=w199, "data path"=w211, "ADCintercadr_s"=w179) -> (w210:T6)
          n124 = case shown="False" w213 {
            tunnel: w234 -> [_ w294]
            tunnel: [w291 w293] -> w223
            tunnel: w233 -> [w291 w292]
            frame False {
            }
            frame True {
              n125 = Divide(x=w292, y=w294) -> (x/y=w293:dbl[])
            }
          }
          n126 = Reciprocal(x=w206) -> (1/x=w205:dbl)
          n127 = Multiply(x=w205, y=w176) -> (x*y=w224:dbl)
          n128 = To Time Stamp(1:w224) -> (0:w225:timestamp)
          n129 = Bundle By Name("Y"=w223, "dt"=w179, "t0"=w225) -> (w221:waveform(dbl))  [unwired: 1 in]
          n130 = Set Waveform Attribute(4:w222, 5:w210, 6:"info" ("name"), 7:w221) -> (0:w226:errorcluster, 3:w209:waveform(dbl))  [unwired: 1 out]
          n131 = case shown="3" w192 {
            tunnel: w209 -> [w238 w242 w254 w288]
            tunnel: [w238 w241 w245 w290] -> w212
            tunnel: w226 -> [w239 w240 w253 w289]
            tunnel: [w239 w240 w244 w289] -> w220
            tunnel: w178 -> [_ _ _ w284]
            tunnel: w177 -> [_ _ _ w283]
            tunnel: w176 -> [_ _ _ w280]
            frame 0, Default {
            }
            frame 1 {
              w243 = 0.0025  # 5(V)/2000(adc)
              n132 = Multiply(x=w242, y=w243) -> (x*y=w241:waveform(dbl))
            }
            frame 2 {
              n133 = call-poly <vilib>:"Number of Waveform Samples.vi"("error in (no error)"=w253, "waveform in"=w254) -> ("error out"=w244:errorcluster, "number of samples"=w252:i32, "waveform out"=w246:waveform(dbl))  [unwired: 7 in]
              n134 = Unbundle By Name(w246) -> ("Y"=w251:dbl[])
              n135 = Divide(x=5.12, y=2048.0) -> (x/y=w248:dbl)
              n136 = for {
                N: w252 -> [_]
                tunnel: w251 -> [w276]
                tunnel: w248 -> [w258]
                tunnel: [w255] -> w247 mode=indexing
                i -> [w275]
                n137 = Index Array(array=w276, index=w275) -> (element=w261:dbl)
                n138 = Subtract(x=w261, y=1.0) -> (x-y=w269:dbl)
                n139 = Add(x=w261, y=4095.0) -> (x+y=w259:dbl)
                n140 = Greater Or Equal?(x=w261, y=i16 -2046) -> (x >= y?=w274:bool)
                n141 = Less Or Equal?(x=w261, y=i16 -2047 ("length")) -> (x <= y?=w268:bool)
                n142 = Greater Or Equal?(x=w261, y=i16 -4095) -> (x >= y?=w267:bool)
                n143 = Multiply(x=w258, y=w269) -> (x*y=w260:dbl)
                n144 = Less Or Equal?(x=w261, y=i16 -1 ("length")) -> (x <= y?=w277:bool)
                n145 = Multiply(x=w259, y=w258) -> (x*y=w257:dbl)
                n146 = And(x=w277, y=w274) -> (x .and. y?=w270:bool)
                n147 = And(x=w268, y=w267) -> (x .and. y?=w264:bool)
                n148 = Select(t=w257, s=w264, f=0.0) -> (s? t:f=w263:dbl)
                n149 = Select(t=w260, s=w270, f=w263) -> (s? t:f=w255:dbl)
              }
              n150 = Bundle By Name(cluster=w246, "Y"=w247) -> (w245:waveform(dbl))
            }
            frame 3 {
              w282 = u16 0 items=["3000mV", "1000mV", "300mV"]  # ADC_INPUT_RANGES_E2010
              w285 = 0.000405  # 3.31776(V)/8192(adc)
              (unwired) 0.0004074  # 3.337(V)/8191(adc)
              n151 = Add(x=w282, y=w280) -> (x+y=w279:i32)
              n152 = Index Array "adc_scale"(array=w284, index=w279) -> ()  [unwired: 1 out]
              n153 = Index Array "adc_offset"(array=w283, index=w279) -> (element=w281:dbl)
              n154 = Add(x=w288, y=w281) -> (x+y=w287:waveform(dbl))
              n155 = Multiply(x=w287, y=1.0) -> (x*y=w286:waveform(dbl))
              n156 = Multiply(x=w286, y=w285) -> (x*y=w290:waveform(dbl))
            }
          }
        }
      }
      n157 = Bundle(w123, w122) -> (w121:cluster{string[], waveform(dbl)[]})  [unwired: 1 in]
    }
    frame True {
      n158 = property on="txt data rate, Hz" class="Arr (strict)"() -> ("Value"=w370:dbl[])  [unwired: 2 in, 2 out]
      n159 = call "txt reader.vi"("data info template"=w372, "error in (no error)"=w375, "sampling rate, Hz"=w370, "file paths"=w376, "how many files"=w377) -> ("error out"=w374:errorcluster, "source txt"=w373:T1, "channels quantity in file"=w371:i32[])  [unwired: 3 in, 1 out]
    }
  }
  "error out" <- w27
  "source" <- w19
  "chan.in.files" <- w17
